vi "KB-Collect Data Judge.vi"(8 "ALL Tolerance Param":string[][](table)=[["Null", "Null", "Null", "Null", "Null", "Null", "Null", "Null", "Null"], ["Null", "Null", "Null", "Null", "Null", "Null", "Null", "Null", "Null"], ["Null", "Null", "Null", "Null", "Null", "Null", "Null", "Null", "Null"], ["Null", "Null", "Null", "Null", "Null", "Null", "Null", "Null", "Null"], ["Null", "Null", "Null", "Null", "Null", "Null", "Null", "Null", "Null"], ["Null", "Null", "Null", "Null", "Null", "Null", "Null", "Null", "Null"], ["Null", "Null", "Null", "Null", "Null", "Null", "Null", "Null", "Null"], ["Null", "Null", "Null", "Null", "Null", "Null", "Null", "Null", "Null"], ["Null", "Null", "Null", "Null", "Null", "Null", "Null", "Null", "Null"], ["Null", "Null", "Null", "Null", "Null", "Null", "Null", "Null", "Null"], ["Null", "Null", "Null", "Null", "Null", "Null", "Null", "Null", "Null"], ["Null", "Null", "Null", "Null", "Null", "Null", "Null", "Null", "Null"], ["Null", "Null", "Null", "Null", "Null", "Null", "Null", "Null", "Null"], ["Null", "Null", "Null", "Null", "Null", "Null", "Null", "Null", "Null"], ["Null", "Null", "Null", "Null", "Null", "Null", "Null", "Null", "Null"], ["Null", "Null", "Null", "Null", "Null", "Null", "Null", "Null", "Null"], ["Null", "Null", "Null", "Null", "Null", "Null", "Null", "Null", "Null"], ["Null", "Null", "Null", "Null", "Null", "Null", "Null", "Null", "Null"], ["Null", "Null", "Null", "Null", "Null", "Null", "Null", "Null", "Null"], ["Null", "Null", "Null", "Null", "Null", "Null", "Null", "Null", "Null"], ["Null", "Null", "Null", "Null", "Null", "Null", "Null", "Null", "Null"], ["Null", "Null", "Null", "Null", "Null", "Null", "Null", "Null", "Null"], ["Null", "Null", "Null", "Null", "Null", "Null", "Null", "Null", "Null"], ["Null", "Null", "Null", "Null", "Null", "Null", "Null", "Null", "Null"], ["Null", "Null", "Null", "Null", "Null", "Null", "Null", "Null", "Null"], ["Null", "Null", "Null", "Null", "Null", "Null", "Null", "Null", "Null"], ["Null", "Null", "Null", "Null", "Null", "Null", "Null", "Null", "Null"], ["Null", "Null", "Null", "Null", "Null", "Null", "Null", "Null", "Null"], ["Null", "Null", "Null", "Null", "Null", "Null", "Null", "Null", "Null"], ["Null", "Null", "Null", "Null", "Null", "Null", "Null", "Null", "Null"], ["Null", "Null", "Null", "Null", "Null", "Null", "Null", "Null", "Null"], ["Null", "Null", "Null", "Null", "Null", "Null", "Null", "Null", "Null"], ["Null", "Null", "Null", "Null", "Null", "Null", "Null", "Null", "Null"]], 11 "Data Result":string[][](table)) -> (3 "Data Result 2":string[][](table))   [LabVIEW 2015]
panel:
  out "转置的数组":string[][](array[string])
  out "Data Result 3":string[](array[string])
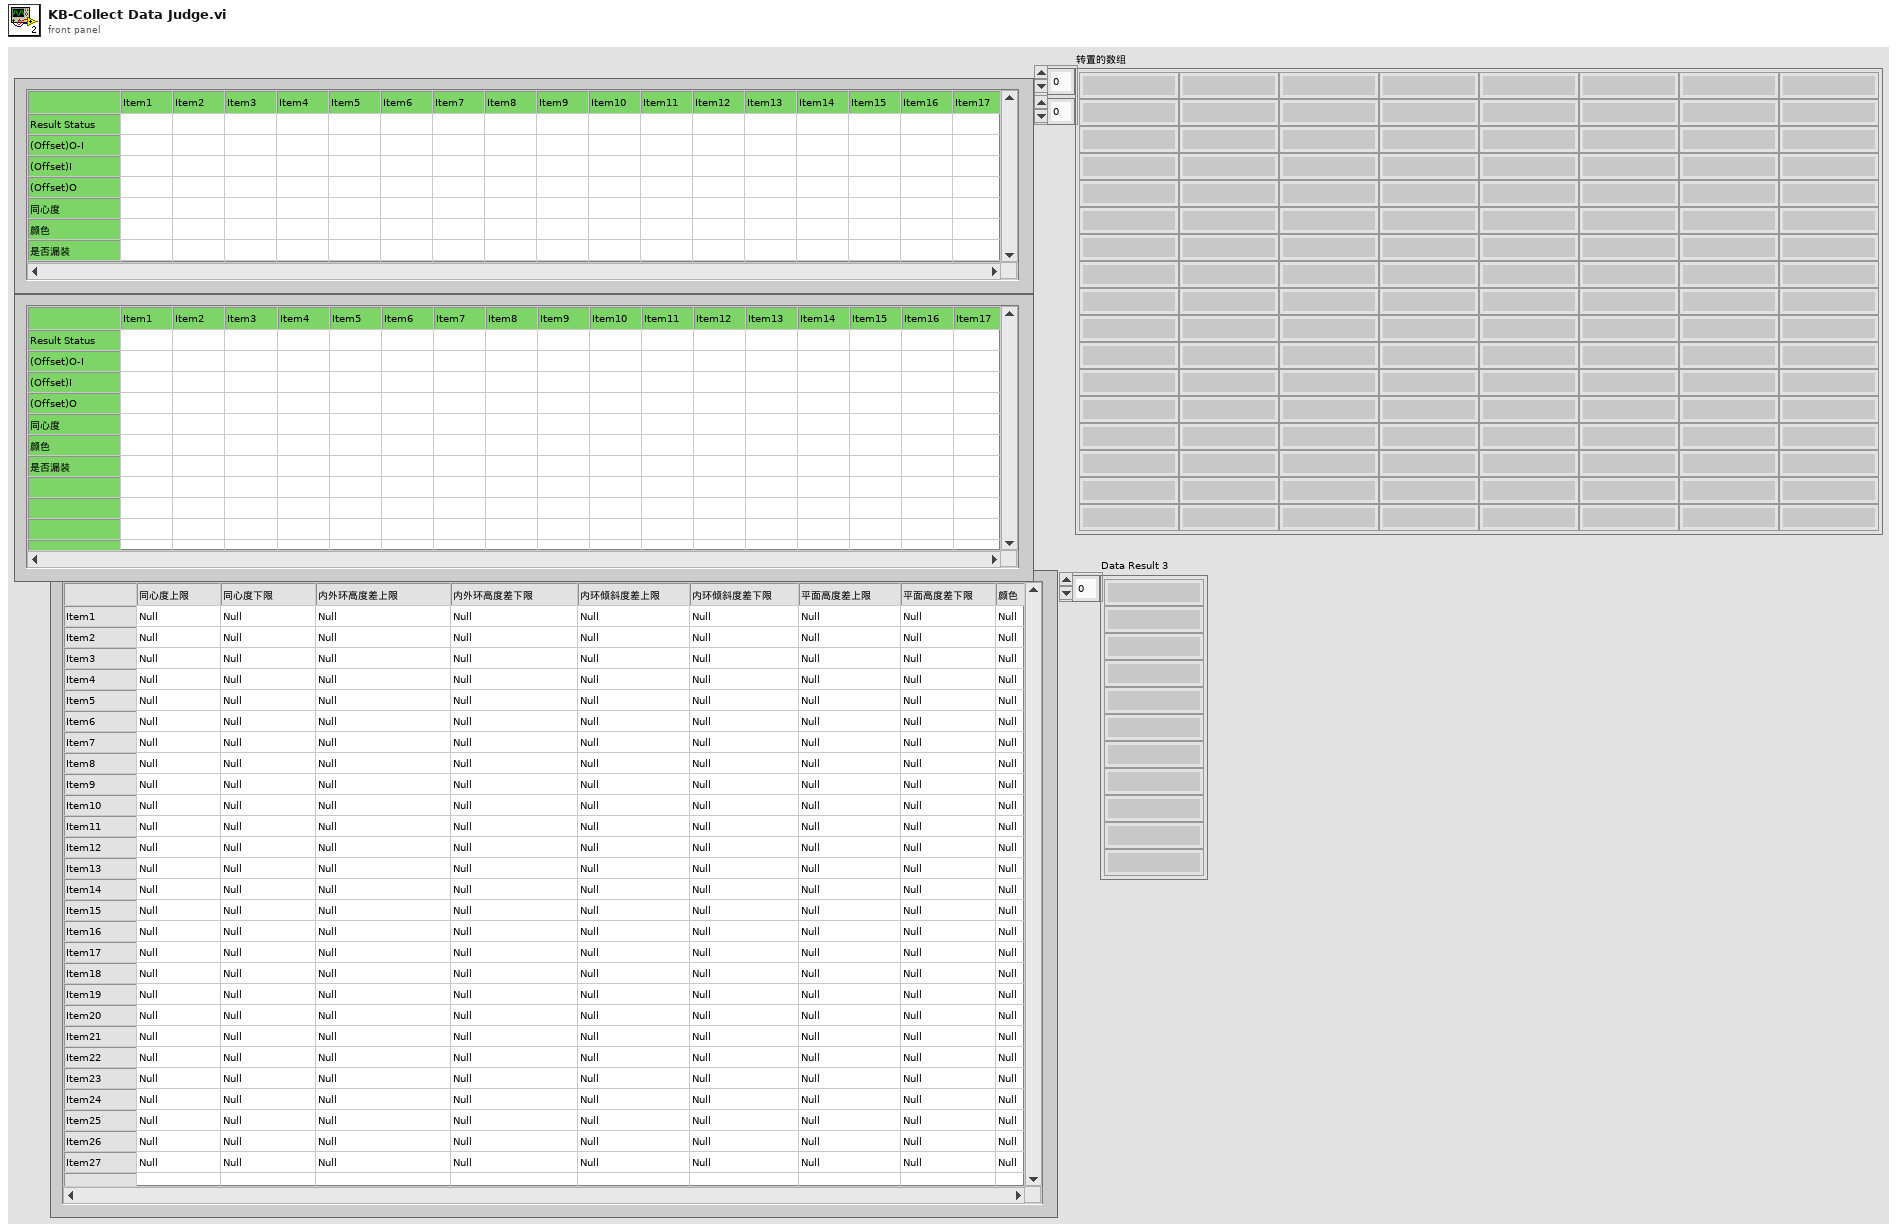
[diagram p1: front panel]
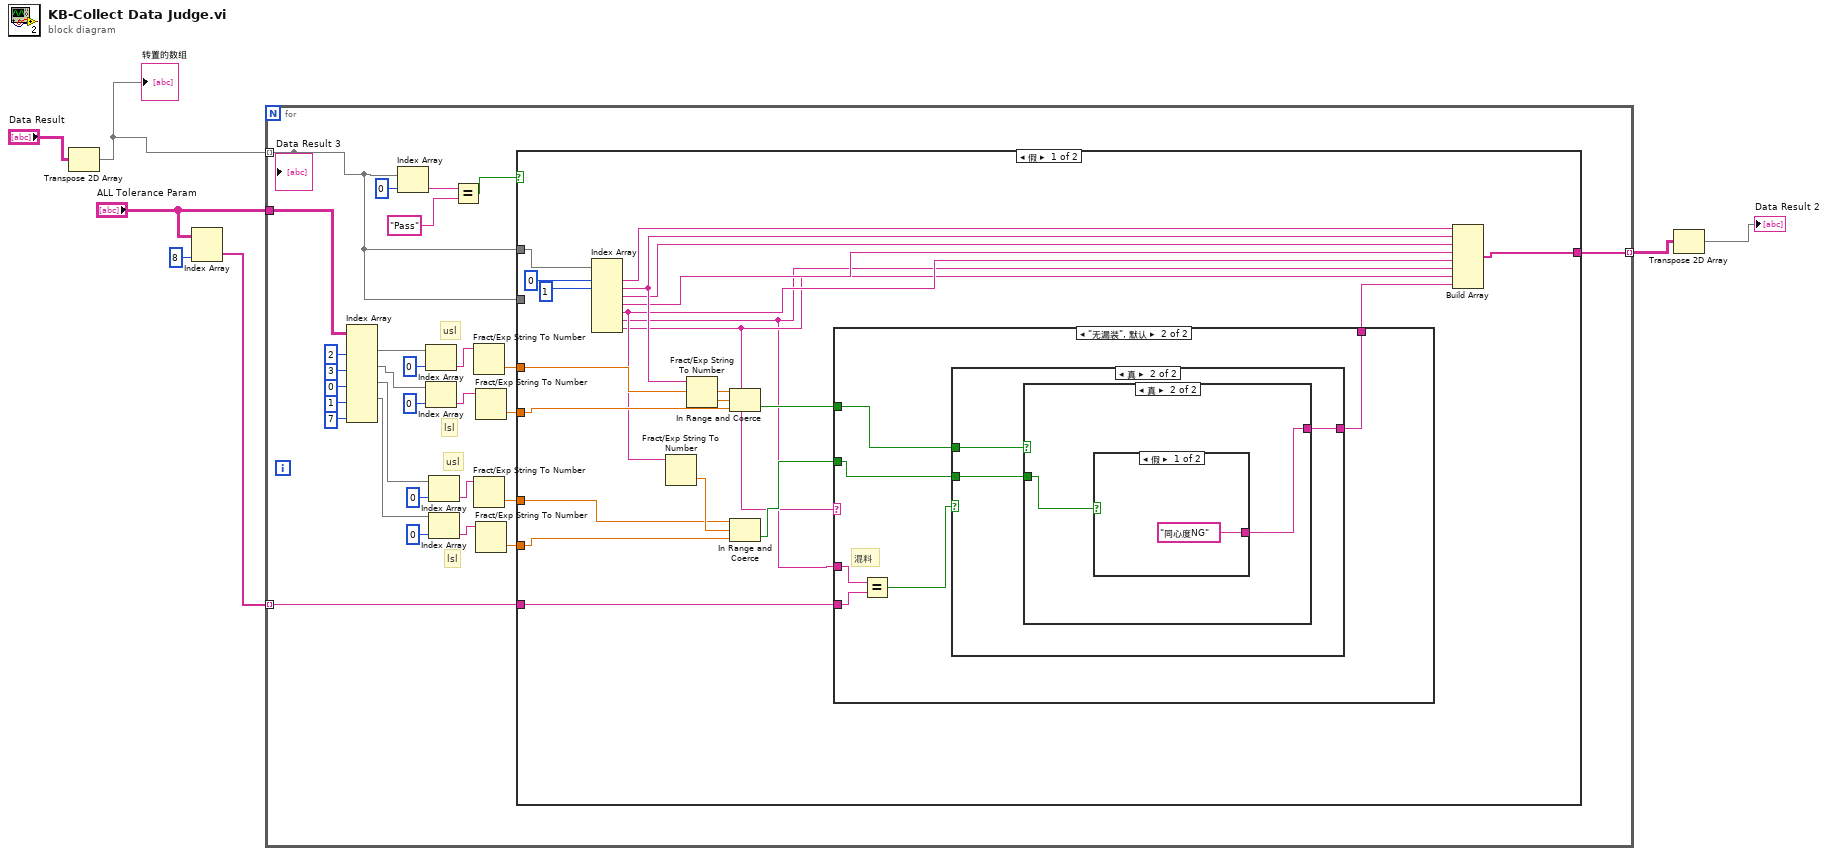
[diagram p0: block diagram]
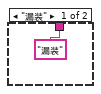
[diagram p2: hidden frame]
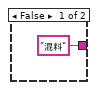
[diagram p3: hidden frame]
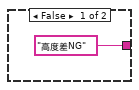
[diagram p4: hidden frame]
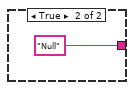
[diagram p5: hidden frame]
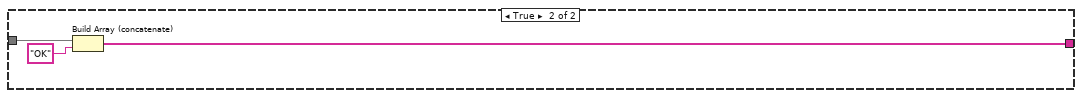
[diagram p6: hidden frame]
diagram:
  n1 = Transpose 2D Array(2D array="Data Result") -> (transposed array=w4:string[][])
  "转置的数组" <- w4
  n2 = Index Array(array="ALL Tolerance Param", index (col)=8 ("禁用的索引 (列)")) -> (element=w1:string[])  [unwired: 1 in]
  n3 = for {
    tunnel: w4 -> [w10] mode=indexing
    tunnel: "ALL Tolerance Param" -> [w31]
    tunnel: [w32] -> w7 mode=indexing
    tunnel: w1 -> [w8] mode=indexing
    # "lsl"
    # "usl"
    # "lsl"
    # "usl"
    n4 = Index Array(array=w31, index (col) #1=2 ("禁用的索引 (列)"), index (col) #2=3 ("索引 (列)"), index (col) #3=0 ("索引 (列)"), index (col) #4=1 ("索引 (列)"), index (col) #5=7 ("索引 (列)")) -> (element #1=w28:string[], element #2=w25:string[], element #3=w16:string[], element #4=w15:string[])  [unwired: 5 in, 1 out]
    n5 = Index Array(array=w10, index=0 ("索引")) -> (element=w35:string)
    n6 = Index Array(array=w28, index=0 ("索引")) -> (element=w24:string)
    n7 = Index Array(array=w25, index=0 ("索引")) -> (element=w23:string)
    n8 = Index Array(array=w16, index=0 ("索引")) -> (element=w14:string)
    n9 = Index Array(array=w15, index=0 ("索引")) -> (element=w13:string)
    n10 = Equal?(x=w35, y="Pass") -> (x = y?=w33:bool)
    n11 = Fract/Exp String To Number(string=w24) -> (number=w22:dbl)  [unwired: 3 in, 1 out]
    n12 = Fract/Exp String To Number(string=w14) -> (number=w12:dbl)  [unwired: 3 in, 1 out]
    n13 = Fract/Exp String To Number(string=w23) -> (number=w21:dbl)  [unwired: 3 in, 1 out]
    n14 = Fract/Exp String To Number(string=w13) -> (number=w11:dbl)  [unwired: 3 in, 1 out]
    n15 = case shown="假" w33 {
      tunnel: w10 -> [w57 w76]
      tunnel: [w47 w74] -> w32
      tunnel: w10 -> [_ _]
      tunnel: w22 -> [w53 _]
      tunnel: w21 -> [w52 _]
      tunnel: w12 -> [w44 _]
      tunnel: w11 -> [w43 _]
      tunnel: w8 -> [w37 _]
      frame False {
        n16 = Index Array(array=w57, index #1=0 ("索引"), index #2=1 ("索引")) -> (element #1=w51:string, element #2=w50:string, element #3=w49:string, element #4=w48:string, element #5=w46:string, element #6=w38:string, element #7=w39:string)  [unwired: 5 in]
        n17 = Fract/Exp String To Number(string=w46) -> (number=w45:dbl)  [unwired: 3 in, 1 out]
        n18 = Fract/Exp String To Number(string=w50) -> (number=w54:dbl)  [unwired: 3 in, 1 out]
        n19 = In Range and Coerce(upper limit=w53, x=w54, lower limit=w52) -> (In Range?=w42:bool)  [unwired: 1 out]
        n20 = In Range and Coerce(upper limit=w44, x=w45, lower limit=w43) -> (In Range?=w40:bool)  [unwired: 1 out]
        n21 = case shown="\"无漏装\", 默认" w39 {
          tunnel: w42 -> [_ w64]
          tunnel: ["漏装" w63] -> w41
          tunnel: w40 -> [_ w62]
          tunnel: w38 -> [_ w61]
          tunnel: w37 -> [_ w60]
          frame "漏装" {
          }
          frame "无漏装", Default {
            # "混料"
            n22 = Equal?(x=w61, y=w60) -> (x = y?=w59:bool)
            n23 = case shown="真" w59 {
              tunnel: w64 -> [_ w68]
              tunnel: ["混料" w67] -> w63
              tunnel: w62 -> [_ w66]
              frame False {
              }
              frame True {
                n24 = case shown="真" w68 {
                  tunnel: ["高度差NG" w70] -> w67
                  tunnel: w66 -> [_ w71]
                  frame False {
                  }
                  frame True {
                    n25 = case shown="假" w71 {
                      tunnel: ["同心度NG" "Null"] -> w70
                      frame False {
                      }
                      frame True {
                      }
                    }
                  }
                }
              }
            }
          }
        }
        n26 = Build Array(w51, w50, w49, w48, w46, w38, w39, w41) -> (w47:string[])
      }
      frame True {
        n27 = Build Array (concatenate)(w76, "OK") -> (w74:string[])
      }
    }
    "Data Result 3" <- w10
  }
  n28 = Transpose 2D Array(2D array=w7) -> (transposed array=→"Data Result 2":string[][])
